vi "globalStimulationPK.vi"() -> ()   [LabVIEW 2011]
uses:
  Database/StimulationPrimary.ctl
panel:
  in  "StimulationPK":T1
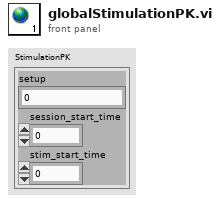
[diagram p1: front panel]
types:
  T1 = typedef "StimulationPrimary.ctl" = cluster{"setup":u8, "session_start_time":dbl, "stim_start_time":dbl}
diagram:
